vi "test_CCDGetSpeedAndGain.vi"(8 "error in":errorcluster) -> (0 "error out":errorcluster, 2 "CCD-gain options":string[](array[string]), 3 "CCD-speed options":string[](array[string]))   [LabVIEW 2023]
uses:
  Classes/CCD/CCD.lvclass
  C:/Projects/Horiba/horiba-labview-sdk/Source/Classes/GenericDevice/GenericDevice.lvclass
  <vilib>/addons/_JKI Toolkits/Caraya/classes/Assert/Assert Not Error.vi
  <vilib>/addons/_JKI Toolkits/Caraya/classes/Assert/Assert Not Equal Value_Variant.vi
  <vilib>/addons/_JKI Toolkits/Caraya/classes/Test/Test.lvclass
  <vilib>/addons/_JKI Toolkits/Caraya/classes/Assert/Assert.lvclass
panel:
  # "Connector Pane"
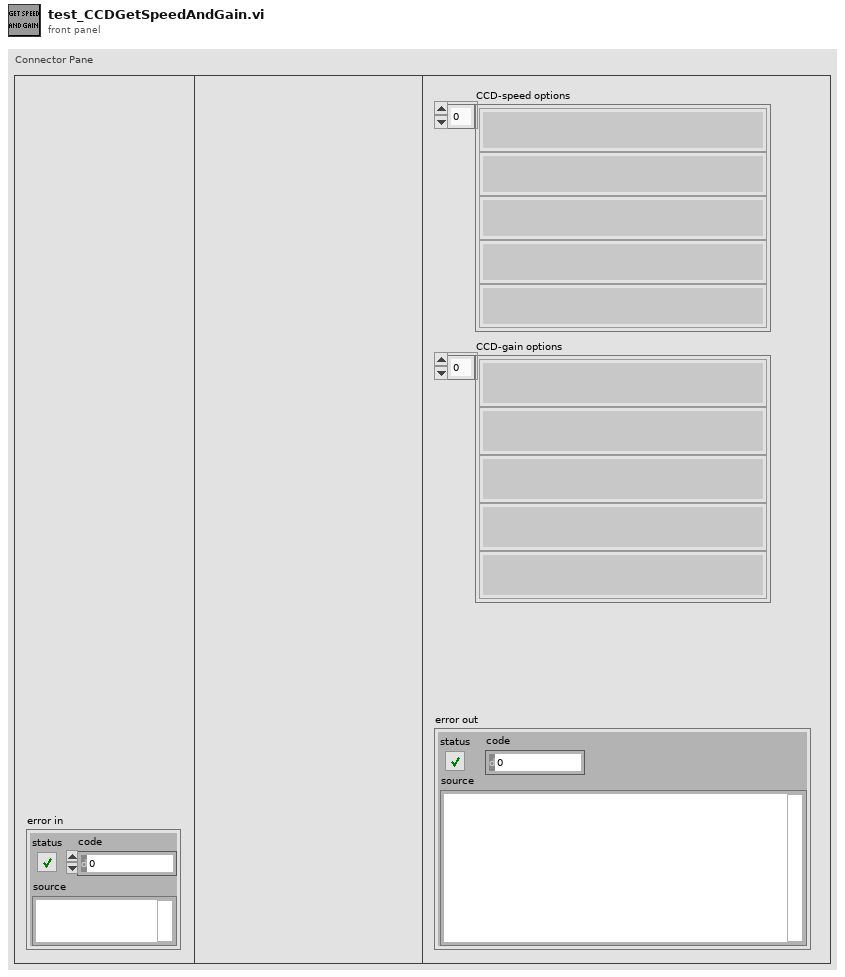
[diagram p1: front panel]
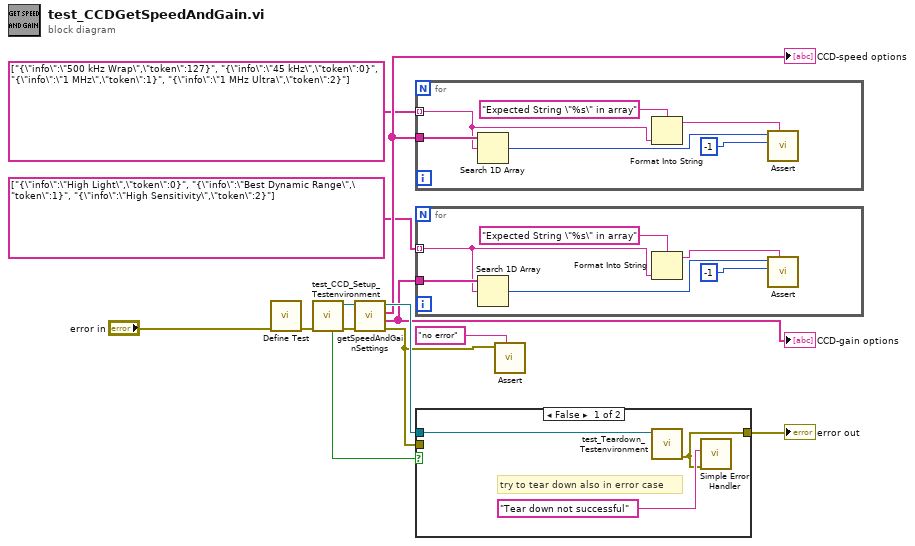
[diagram p0: block diagram]
diagram:
  n1 = call <vilib>:"Define Test.vi"("error in (no error)"="error in") -> ("error out"=w4:errorcluster)  [unwired: 9 in, 1 out]
  n2 = call "test_CCD_Setup_Testenvironment.vi"("error in"=w4) -> ("error out"=w2:errorcluster, "CCD out"=w3:refnum<class "CCD.lvclass">, "Module Was Already Running?"=w1:bool)  [unwired: 7 in, 1 out]
  n3 = call "getSpeedAndGainSettings.vi"("error in (no error)"=w2, "CCD in"=w3) -> ("error out"=w9:errorcluster, "CCD-gain options"=w6:string[], "CCD-speed options"=w8:string[], "CCD out"=w11:refnum<class "CCD.lvclass">)  [unwired: 6 in]
  "CCD-speed options" <- w8
  "CCD-gain options" <- w6
  n4 = for {
    tunnel: w8 -> [w19]
    tunnel: string[] ["{\"info\":\"500 kHz Wrap\",\"token\":127}", "{\"info\":\"45 kHz\",\"token\":0}", "{\"info\":\"1 MHz\",\"token\":1}", "{\"info\":\"1 MHz Ultra\",\"token\":2}"] ("CCD-speed options") -> [w15] mode=indexing
    n5 = Search 1D Array(1D array=w19, element=w15) -> (index of element=w18:i32)  [unwired: 1 in]
    n6 = Format Into String(format string="Expected String \"%s\" in array", w15) -> (resulting string=w14:string)  [unwired: 2 in, 1 out]
    n7 = call-poly <vilib>:"Assert.vi"("Label"=w14, "Y"=-1 ("index of element"), "X"=w18) -> ()  [unwired: 7 in, 2 out]
  }
  n8 = for {
    tunnel: w6 -> [w25]
    tunnel: string[] ["{\"info\":\"High Light\",\"token\":0}", "{\"info\":\"Best Dynamic Range\",\"token\":1}", "{\"info\":\"High Sensitivity\",\"token\":2}"] ("CCD-gain options") -> [w21] mode=indexing
    n9 = Search 1D Array(1D array=w25, element=w21) -> (index of element=w24:i32)  [unwired: 1 in]
    n10 = Format Into String(format string="Expected String \"%s\" in array", w21) -> (resulting string=w20:string)  [unwired: 2 in, 1 out]
    n11 = call-poly <vilib>:"Assert.vi"("Label"=w20, "Y"=-1 ("index of element"), "X"=w24) -> ()  [unwired: 7 in, 2 out]
  }
  n12 = case shown="False" w1 {
    tunnel: w11 -> [w27 _]
    tunnel: [w26 w29] -> w10
    tunnel: w9 -> [_ w29]
    frame False {
      # "try to tear down also in error case"
      n13 = call "test_Teardown_Testenvironment.vi"("GenericDevice.lvclass"=w27) -> ("error out"=w26:errorcluster)  [unwired: 9 in, 1 out]
      n14 = call <vilib>:"Simple Error Handler.vi"("error source (\" \")"="Tear down not successful" ("error source (\" \")"), "error in (no error)"=w26) -> ()  [unwired: 3 in, 5 out]
    }
    frame True {
    }
  }
  "error out" <- w10
  n15 = call-poly <vilib>:"Assert.vi"("Label"="no error" ("Label (VI Title)"), "Not Error?"=w9) -> ()  [unwired: 8 in, 2 out]
